vi "Config.vi"() -> (0 "Tolerancia %":sgl, 1 "Delay Auto-Refresh(uS)":i32, 2 "Numero de Tramas - Sequence":i32, 3 "Seleccion de Puerto COM":refnum<visa-resource-name>, 4 "Pulsos Encoder":u16=1, 6 "Delay Sequence(uS)":i32)   [LabVIEW 2014, in "CAP-USB.lvlib"]
uses:
  CAP-USB.lvlib
panel:
  in  "Delay Sequence(uS)":i32
  in  "Pulsos Encoder":u16=3600
  in  "OK Button":bool
  in  "Tolerancia %":sgl=10.0
  in  "N° Tramas - Sequence":i32=90
  in  "Delay Auto-Refresh(uS)":i32=35000
  in  "Seleccion de Puerto COM":refnum<visa-resource-name>="COM3"
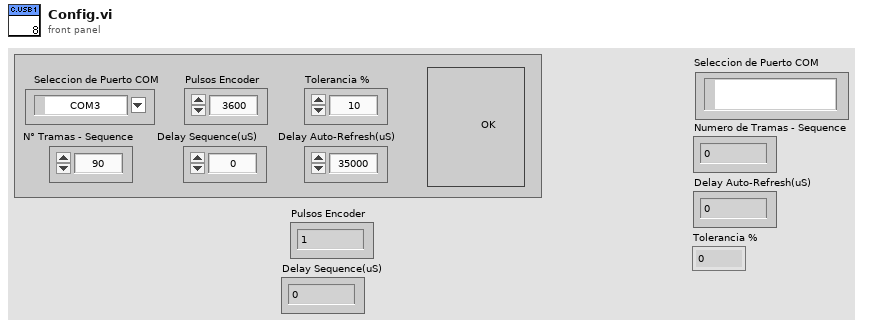
[diagram p1: front panel]
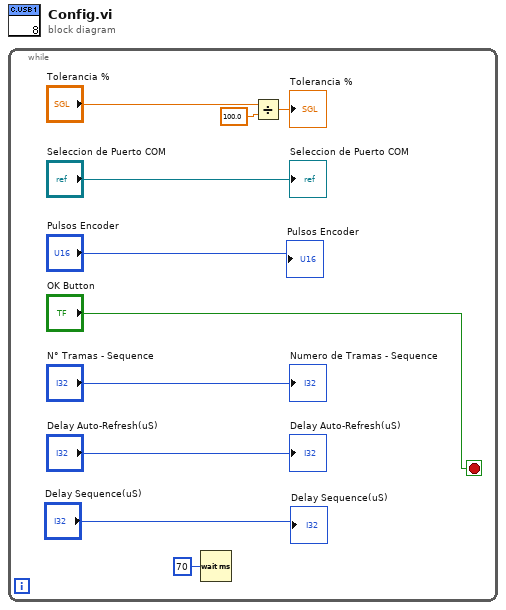
[diagram p0: block diagram]
diagram:
  n1 = while {
    stop <- "OK Button" stop-if-true
    n2 = Wait (ms)(milliseconds to wait=u32 70) -> ()  [unwired: 1 out]
    n3 = Divide(x="Tolerancia %", y=sgl 100.0) -> (x/y=→"Tolerancia %":sgl)
    "Numero de Tramas - Sequence" <- "N° Tramas - Sequence"
    "Delay Auto-Refresh(uS)" <- "Delay Auto-Refresh(uS)"
    "Seleccion de Puerto COM" <- "Seleccion de Puerto COM"
    "Pulsos Encoder" <- "Pulsos Encoder"
    "Delay Sequence(uS)" <- "Delay Sequence(uS)"
  }
